vi "make_axes_labels.vi"(7 "Labels Properties":T7, 8 "length":sgl, 9 "View Direction":T1(ring), 10 "Axis output cluster":T3, 11 "Scene Object In":refnum<vi>) -> (2 "Label Width":T2, 3 "Scene Object Out":refnum<vi>)   [LabVIEW 2020, in "3DPC_SurfacePlot.xctl"]
uses:
  <vilib>/Native 3D Graph/xcontrol/3DPC_SurfacePlot.xctl
  <vilib>/Native 3D Graph/typedefs/prop_axes_labels.ctl
  <vilib>/Native 3D Graph/typedefs/prop_axes_merged_array_etc.ctl
  <vilib>/Native 3D Graph/typedefs/prop_axes_merged_array.ctl
  <vilib>/Native 3D Graph/typedefs/range_cluster.ctl
  <vilib>/Native 3D Graph/typedefs/min_max.ctl
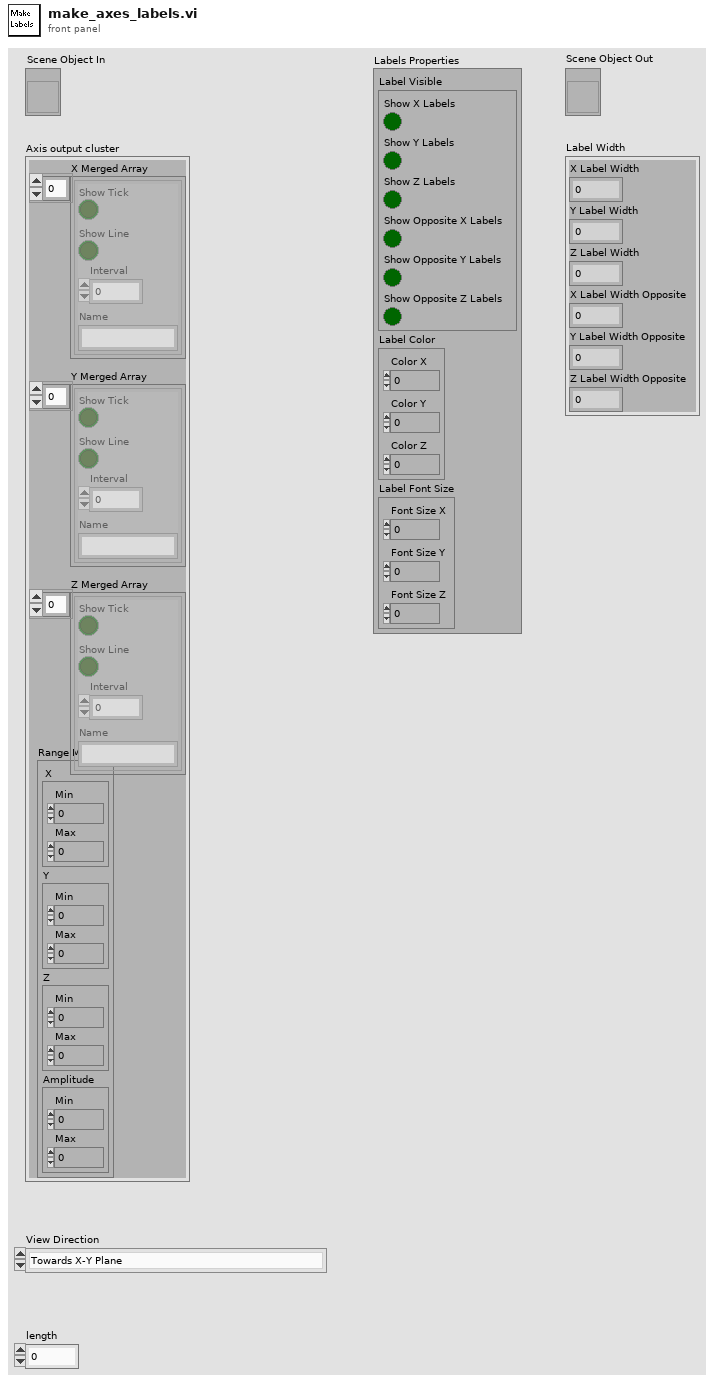
[diagram p1: front panel]
types:
  T1 = enum32{"Towards X-Y Plane", "Towards Y-Z Plane", "Towards X-Z Plane", "User Define"}
  T2 = cluster{"X Label Width":dbl, "Y Label Width":dbl, "Z Label Width":dbl, "X Label Width Opposite":dbl, "Y Label Width Opposite":dbl, "Z Label Width Opposite":dbl}
  T3 = typedef "3DPC_SurfacePlot.xctl/prop_axes_merged_array_etc.ctl" = cluster{"X Merged Array":T4, "Y Merged Array":T4, "Z Merged Array":T4, "Range Min/Max":T5}
  T4 = typedef "3DPC_SurfacePlot.xctl/prop_axes_merged_array.ctl" = cluster{"Show Tick":bool, "Show Line":bool, "Interval":sgl, "Name":string}[]
  T5 = typedef "3DPC_SurfacePlot.xctl/range_cluster.ctl" = cluster{"X":T6, "Y":T6, "Z":T6, "Amplitude":T6}
  T6 = typedef "3DPC_SurfacePlot.xctl/min_max.ctl" = cluster{"Min":sgl, "Max":sgl}
  T7 = typedef "3DPC_SurfacePlot.xctl/prop_axes_labels.ctl" = cluster{"Label Visible":cluster{"Show X Labels":bool, "Show Y Labels":bool, "Show Z Labels":bool, "Show Opposite X Labels":bool, "Show Opposite Y Labels":bool, "Show Opposite Z Labels":bool}, "Label Color":cluster{"Color X":u32, "Color Y":u32, "Color Z":u32}, "Label Font Size":cluster{"Font Size X":i16, "Font Size Y":i16, "Font Size Z":i16}}
  T8 = cluster{"Show X Labels":bool, "Show Y Labels":bool, "Show Z Labels":bool, "Show Opposite X Labels":bool, "Show Opposite Y Labels":bool, "Show Opposite Z Labels":bool}
  T9 = enum16{"X", "Y", "Z", "X Opposite", "Y Opposite", "Z Opposite"}
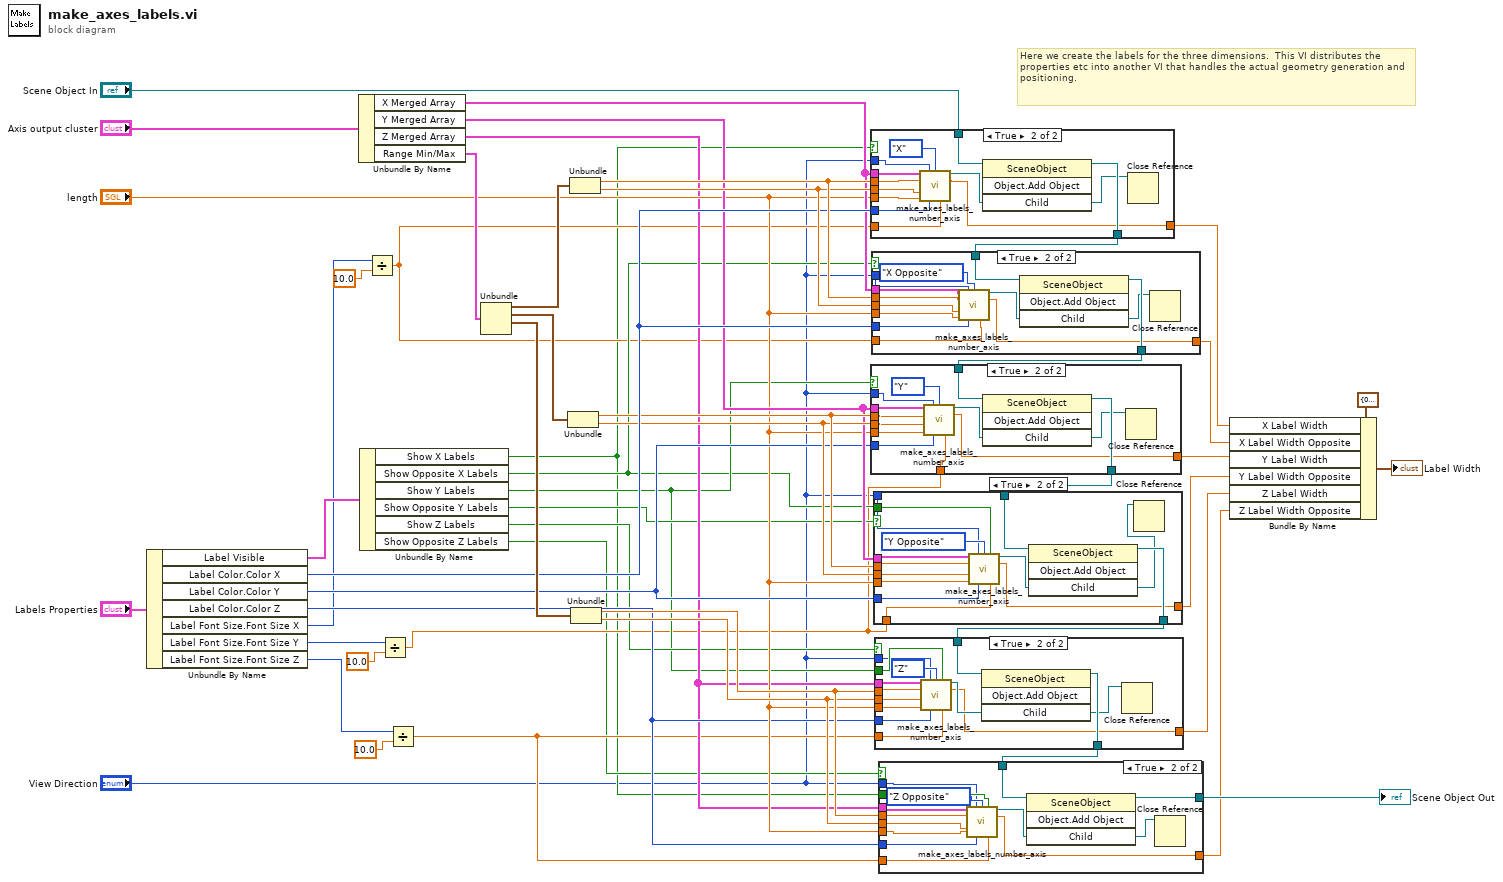
[diagram p0: block diagram]
diagram:
  # "Here we create the labels for the three dimensions.  This VI distributes the properties etc into another VI that handles the actual geometry generation and positioning."
  n1 = Unbundle By Name("Labels Properties") -> ("Label Visible"=w14:T8, "Label Color.Color X"=w41:u32, "Label Color.Color Y"=w33:u32, "Label Color.Color Z"=w27:u32, "Label Font Size.Font Size X"=w11:i16, "Label Font Size.Font Size Y"=w8:i16, "Label Font Size.Font Size Z"=w5:i16)
  n2 = Unbundle By Name("Axis output cluster") -> ("X Merged Array"=w40:T4, "Y Merged Array"=w34:T4, "Z Merged Array"=w26:T4, "Range Min/Max"=w45:T5)
  n3 = Unbundle By Name(w14) -> ("Show X Labels"=w2:bool, "Show Opposite X Labels"=w13:bool, "Show Y Labels"=w15:bool, "Show Opposite Y Labels"=w17:bool, "Show Z Labels"=w16:bool, "Show Opposite Z Labels"=w3:bool)
  n4 = Divide(x=w11, y=10.0) -> (x/y=w10:dbl)
  n5 = Divide(x=w8, y=10.0) -> (x/y=w7:dbl)
  n6 = Divide(x=w5, y=10.0) -> (x/y=w4:dbl)
  n7 = Unbundle(w45) -> ("X"=w50:T6, "Y"=w49:T6, "Z"=w48:T6)  [unwired: 1 out]
  n8 = Unbundle(w49) -> ("Min"=w36:sgl, "Max"=w35:sgl)
  n9 = Unbundle(w50) -> ("Min"=w43:sgl, "Max"=w42:sgl)
  n10 = Unbundle(w48) -> ("Min"=w30:sgl, "Max"=w29:sgl)
  n11 = case shown="True" w2 {
    tunnel: "Scene Object In" -> [w52 w65]
    tunnel: [w52 w64] -> w44
    tunnel: w43 -> [_ w58]
    tunnel: w42 -> [_ w59]
    tunnel: w41 -> [_ w61]
    tunnel: "length" -> [_ w60]
    tunnel: [_ w54] -> w23
    tunnel: w40 -> [_ w57]
    tunnel: w10 -> [_ w62]
    tunnel: "View Direction" -> [_ w55]
    frame False {
    }
    frame True {
      n12 = call <vilib>:"make_axes_labels_number_axis.vi"("Merged Array Out"=w57, "View Direction"=w55, "Which Axis?"=T9."X", "from"=w58, "to"=w59, "axis-offset"=w60, "Font Color"=w61, "Font Size"=w62) -> ("Scene:New Object"=w53:refnum<vi>, "Max Width"=w54:dbl)  [unwired: 1 in, 5 out]
      n13 = invoke class="SceneObject" method="Object.Add Object"(reference=w65, "Child"=w53) -> (reference out=w64:refnum<vi>, "Child"=w63:refnum<vi>)  [unwired: 2 in, 2 out]
      n14 = Close Reference(reference=w63) -> ()  [unwired: 1 in, 1 out]
    }
  }
  n15 = case shown="True" w13 {
    tunnel: w44 -> [w66 w79]
    tunnel: [w66 w78] -> w39
    tunnel: w43 -> [_ w71]
    tunnel: w42 -> [_ w72]
    tunnel: w41 -> [_ w74]
    tunnel: "length" -> [_ w73]
    tunnel: [_ w67] -> w22
    tunnel: w40 -> [_ w70]
    tunnel: w10 -> [_ w75]
    tunnel: "View Direction" -> [_ w69]
    frame False {
    }
    frame True {
      n16 = call <vilib>:"make_axes_labels_number_axis.vi"("Merged Array Out"=w70, "View Direction"=w69, "Which Axis?"=T9."X Opposite", "from"=w71, "to"=w72, "axis-offset"=w73, "Font Color"=w74, "Font Size"=w75) -> ("Scene:New Object"=w68:refnum<vi>, "Max Width"=w67:dbl)  [unwired: 1 in, 5 out]
      n17 = invoke class="SceneObject" method="Object.Add Object"(reference=w79, "Child"=w68) -> (reference out=w78:refnum<vi>, "Child"=w77:refnum<vi>)  [unwired: 2 in, 2 out]
      n18 = Close Reference(reference=w77) -> ()  [unwired: 1 in, 1 out]
    }
  }
  n19 = case shown="True" w15 {
    tunnel: w39 -> [w80 w93]
    tunnel: [w80 w92] -> w38
    tunnel: w36 -> [_ w89]
    tunnel: w35 -> [_ w88]
    tunnel: w33 -> [_ w86]
    tunnel: "length" -> [_ w87]
    tunnel: [_ w83] -> w21
    tunnel: w34 -> [_ w90]
    tunnel: w7 -> [_ w85]
    tunnel: "View Direction" -> [_ w81]
    frame False {
    }
    frame True {
      n20 = call <vilib>:"make_axes_labels_number_axis.vi"("Merged Array Out"=w90, "View Direction"=w81, "Which Axis?"=T9."Y", "from"=w89, "to"=w88, "axis-offset"=w87, "Font Color"=w86, "Font Size"=w85) -> ("Scene:New Object"=w84:refnum<vi>, "Max Width"=w83:dbl)  [unwired: 1 in, 5 out]
      n21 = invoke class="SceneObject" method="Object.Add Object"(reference=w93, "Child"=w84) -> (reference out=w92:refnum<vi>, "Child"=w91:refnum<vi>)  [unwired: 2 in, 2 out]
      n22 = Close Reference(reference=w91) -> ()  [unwired: 1 in, 1 out]
    }
  }
  n23 = case shown="True" w17 {
    tunnel: w38 -> [w94 w108]
    tunnel: [w94 w107] -> w37
    tunnel: w36 -> [_ w101]
    tunnel: w35 -> [_ w100]
    tunnel: "length" -> [_ w99]
    tunnel: [_ w95] -> w20
    tunnel: w34 -> [_ w102]
    tunnel: w33 -> [_ w98]
    tunnel: w13 -> [_ w105]
    tunnel: w7 -> [_ w97]
    tunnel: "View Direction" -> [_ w103]
    frame False {
    }
    frame True {
      n24 = call <vilib>:"make_axes_labels_number_axis.vi"("Merged Array Out"=w102, "View Direction"=w103, "Which Axis?"=T9."Y Opposite", "Draw Y?"=w105, "from"=w101, "to"=w100, "axis-offset"=w99, "Font Color"=w98, "Font Size"=w97) -> ("Scene:New Object"=w96:refnum<vi>, "Max Width"=w95:dbl)  [unwired: 5 out]
      n25 = invoke class="SceneObject" method="Object.Add Object"(reference=w108, "Child"=w96) -> (reference out=w107:refnum<vi>, "Child"=w106:refnum<vi>)  [unwired: 2 in, 2 out]
      n26 = Close Reference(reference=w106) -> ()  [unwired: 1 in, 1 out]
    }
  }
  n27 = case shown="True" w16 {
    tunnel: w37 -> [w109 w123]
    tunnel: w30 -> [_ w116]
    tunnel: w29 -> [_ w115]
    tunnel: w27 -> [_ w113]
    tunnel: "length" -> [_ w114]
    tunnel: w15 -> [_ w119]
    tunnel: [_ w110] -> w19
    tunnel: w26 -> [_ w117]
    tunnel: [w109 w122] -> w32
    tunnel: w4 -> [_ w112]
    tunnel: "View Direction" -> [_ w118]
    frame False {
    }
    frame True {
      n28 = call <vilib>:"make_axes_labels_number_axis.vi"("Merged Array Out"=w117, "View Direction"=w118, "Which Axis?"=T9."Z", "Draw Y?"=w119, "from"=w116, "to"=w115, "axis-offset"=w114, "Font Color"=w113, "Font Size"=w112) -> ("Scene:New Object"=w111:refnum<vi>, "Max Width"=w110:dbl)  [unwired: 5 out]
      n29 = invoke class="SceneObject" method="Object.Add Object"(reference=w123, "Child"=w111) -> (reference out=w122:refnum<vi>, "Child"=w121:refnum<vi>)  [unwired: 2 in, 2 out]
      n30 = Close Reference(reference=w121) -> ()  [unwired: 1 in, 1 out]
    }
  }
  n31 = case shown="True" w3 {
    tunnel: w32 -> [w124 w138]
    tunnel: [w124 w137] -> w31
    tunnel: w30 -> [_ w130]
    tunnel: w29 -> [_ w129]
    tunnel: w27 -> [_ w127]
    tunnel: "length" -> [_ w128]
    tunnel: w2 -> [_ w134]
    tunnel: [_ w125] -> w18
    tunnel: w26 -> [_ w131]
    tunnel: w4 -> [_ w126]
    tunnel: "View Direction" -> [_ w132]
    frame False {
    }
    frame True {
      n32 = call <vilib>:"make_axes_labels_number_axis.vi"("Merged Array Out"=w131, "View Direction"=w132, "Which Axis?"=T9."Z Opposite", "Draw Y?"=w134, "from"=w130, "to"=w129, "axis-offset"=w128, "Font Color"=w127, "Font Size"=w126) -> ("Scene:New Object"=w135:refnum<vi>, "Max Width"=w125:dbl)  [unwired: 5 out]
      n33 = invoke class="SceneObject" method="Object.Add Object"(reference=w138, "Child"=w135) -> (reference out=w137:refnum<vi>, "Child"=w136:refnum<vi>)  [unwired: 2 in, 2 out]
      n34 = Close Reference(reference=w136) -> ()  [unwired: 1 in, 1 out]
    }
  }
  "Scene Object Out" <- w31
  n35 = Bundle By Name(cluster=T2 {"X Label Width"=0.0, "Y Label Width"=0.0, "Z Label Width"=0.0, "X Label Width Opposite"=0.0, "Y Label Width Opposite"=0.0, "Z Label Width Opposite"=0.0} ("Label Width"), "X Label Width"=w23, "X Label Width Opposite"=w22, "Y Label Width"=w21, "Y Label Width Opposite"=w20, "Z Label Width"=w19, "Z Label Width Opposite"=w18) -> (→"Label Width":T2)
